vi "Read Element of Intervals.vi"(8 "error in (no error)":errorcluster, 9 "Interval":T2, 11 "Cron in":refnum<class "Cron.lvclass">) -> (0 "error out":errorcluster, 2 "Interval":T1, 3 "Cron out":refnum<class "Cron.lvclass">)   [LabVIEW 2013, in "openCron.lvlib" / "Cron.lvclass"]
uses:
  Cron.lvclass
  Cron Interval -- enum.ctl
  Cron Interval -- cluster.ctl
  Cron.lvclass/Cron.ctl
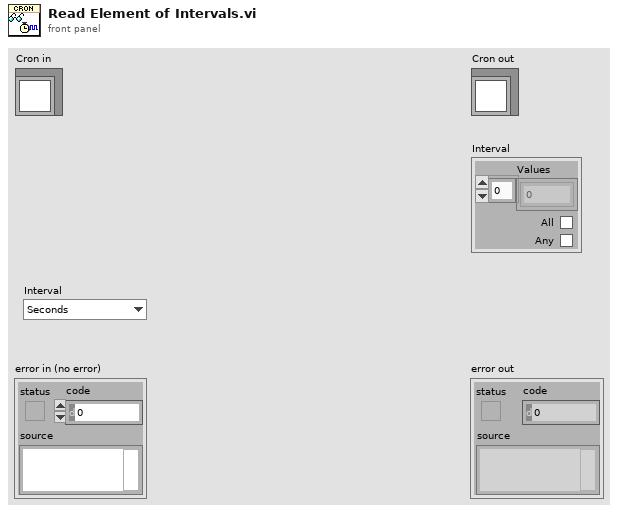
[diagram p1: front panel]
types:
  T1 = typedef "openCron.lvlib/Cron.lvclass/Cron Interval -- cluster.ctl" = cluster{"Values":i32[], "All":bool, "Any":bool}
  T2 = typedef "openCron.lvlib/Cron.lvclass/Cron Interval -- enum.ctl" = enum16{"Seconds", "Minutes", "Hours", "Day of Month", "Month", "Day of Week", "Year"}
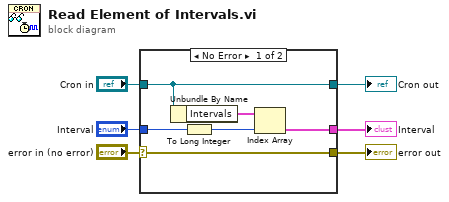
[diagram p0: block diagram]
diagram:
  n1 = case shown="No Error" "error in (no error)" {
    selector: "error in (no error)" -> [w12 w13]
    tunnel: [w12 w13] -> w5
    tunnel: [w11 w14] -> w3
    tunnel: "Cron in" -> [w11 w14]
    tunnel: [w9 _] -> w2
    tunnel: "Interval" -> [w8 _]
    frame No Error {
      n2 = Unbundle By Name(w11) -> ("Intervals"=w10:T1[])
      n3 = To Long Integer(number=w8) -> (32bit integer=w7:i32)
      n4 = Index Array(array=w10, index=w7) -> (element=w9:T1)
    }
    frame Error {
    }
  }
  "error out" <- w5
  "Cron out" <- w3
  "Interval" <- w2
